vi "Team and Side.vi"(5 "Lado":enum16{"Esquerdo", "Direito"}(ring) caption="Enum", 7 "Time":enum16{"Azul", "Amarelo"}(ring) caption="Enum", 9 "Comm RX FPS":dbl, 10 "Game Status":T17 {"Time" format="%<%.3X %x>T"; "Blue Timeout Remaining" format="%<%M:%S>t"; "Yellow Timeout Remaining" format="%<%M:%S>t"; "Time Left" format="%<%M:%S>t"}, 11 "Field State Input":T1 {"Detection Frame Out"."robots_blue"."height" format="%+4.3f"; "Detection Frame Out"."robots_blue"."pixel_y" format="%+4.3f"; "Detection Frame Out"."robots_blue"."pixel_x" format="%+4.3f"; "Detection Frame Out"."robots_blue"."orientation" format="%+4.3f"; "Detection Frame Out"."robots_blue"."y" format="%+4.3f"; "Detection Frame Out"."robots_blue"."confidence" format="%4.3f"; "Detection Frame Out"."robots_blue"."x" format="%+4.3f"; "Detection Frame Out"."robots_yellow"."height" format="%+4.3f"; "Detection Frame Out"."robots_yellow"."pixel_y" format="%+4.3f"; "Detection Frame Out"."robots_yellow"."pixel_x" format="%+4.3f"; "Detection Frame Out"."robots_yellow"."orientation" format="%+4.3f"; "Detection Frame Out"."robots_yellow"."y" format="%+4.3f"; "Detection Frame Out"."robots_yellow"."confidence" format="%4.3f"; "Detection Frame Out"."robots_yellow"."x" format="%+4.3f"}) -> (3 "IA State":T6={"our_robots"=[], "enemy_robots"=[], "balls"=[], "geometry"={"line_width"=0, "field_length"=0, "field_width"=0, "boundary_width"=0, "referee_width"=0, "goal_width"=0, "goal_depth"=0, "goal_wall_width"=0, "center_circle_radius"=0, "defense_radius"=0, "defense_stretch"=0, "free_kick_from_defense_dist"=0, "penalty_spot_from_field_line_dist"=0, "penalty_line_from_spot_dist"=0}, "IA Judge"={"stage"="", "command"="", "our_goalie_id"=0.0, "enemy_goalie_id"=0.0, "command enum"=enum."Halt", "Time"=enum."Azul"}, "Received Timestamp"=timestamp(0 s since 1904-01-01), "Events"={"Touch"=FALSE, "Ball out"=FALSE, "id touch"=0.0, "Ball out of \nVision"=FALSE, "Ball inside \nGoalie area"=FALSE, "Robot not responding"=FALSE, "Robots responding status"=[1.0, 1.0, 1.0, 1.0, 1.0, 1.0], "Enemy Ball \nPossession"=FALSE, "Pass State"=FALSE, "id end of pass"=0.0, "Kick"=FALSE, "Id ini Possession"=0.0, "Ball Possesion"=FALSE, "Id Possesion"=0.0, "Direct Kick"=FALSE, "2nd Strk Ativo"=FALSE}})   [LabVIEW 2018]
uses:
  SSL Referee Game Status.ctl
  Communication_class/Paths/MessageAI_State Folder/Core/AI Input.ctl
  Controls/AI Robot.ctl
  Controls/Functions Enum.ctl
  Controls/AttackerStates.ctl
  Controls/PathDests.ctl
  Controls/PathDest.ctl
  Communication_class/Paths/MessageAI_State Folder/Core/AI Ball.ctl
  Communication_class/Paths/MessageAI_State Folder/Core/Field Size.ctl
  Communication_class/Paths/MessageAI_State Folder/Core/AI Judge.ctl
  Communication_class/Paths/MessageAI_State Folder/Intel/Command Enum.ctl
  Communication_class/Paths/MessageAI_State Folder/Util/Events/Events.ctl
  Controls/SSL Field State.ctl
  Controls/SSL Detection Frame.ctl
  Controls/SSL Detection Robot.ctl
  <vilib>/Analysis/Matrix/Datatypes/RealMatrix.ctl
  Controls/SSL Detection Ball.ctl
  <vilib>/Analysis/Matrix/NI_Matrix.lvlib
panel:
  # "Score"
  # "Red Cards"
  # "Yellow Cards"
  # "Timeouts Left"
  # "Timeout Remaining"
  # "Goalie ID"
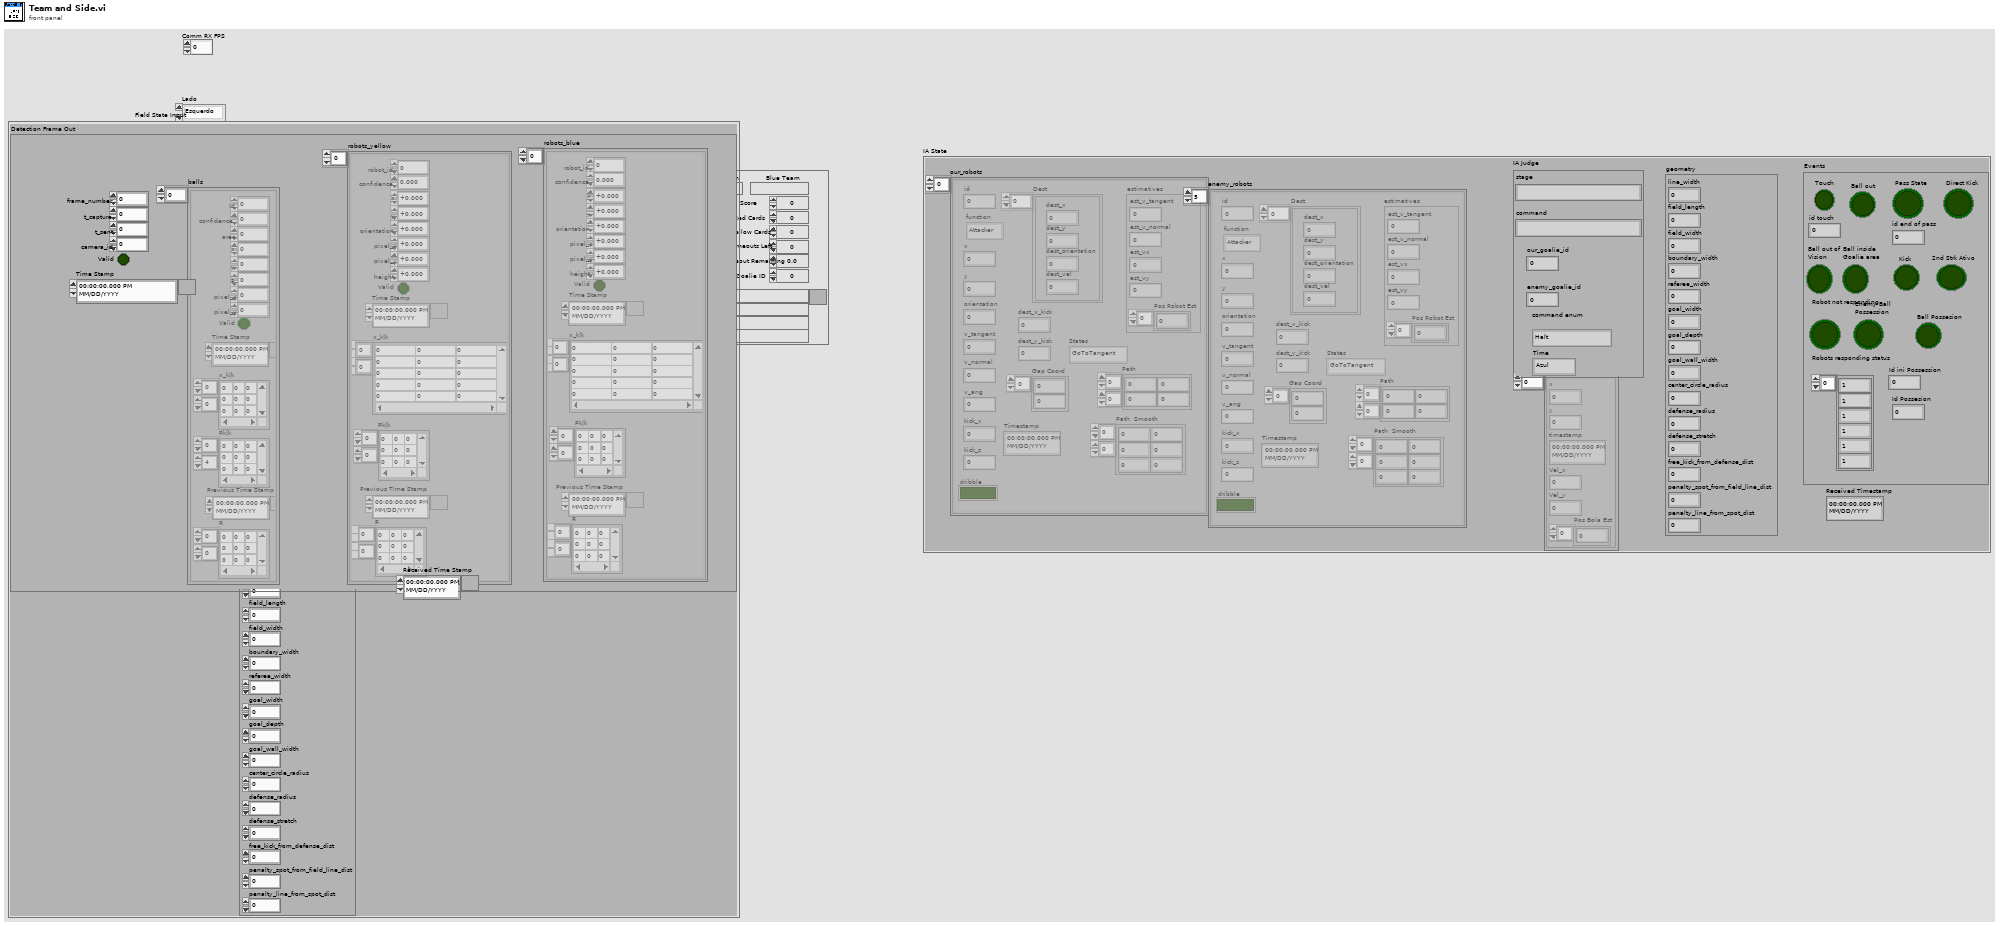
[diagram p1: front panel]
types:
  T1 = typedef "SSL Field State.ctl" = cluster{"Detection Frame Out":T2, "Field Size Out":cluster{"line_width":u32, "field_length":u32, "field_width":u32, "boundary_width":u32, "referee_width":u32, "goal_width":u32, "goal_depth":u32, "goal_wall_width":u32, "center_circle_radius":u32, "defense_radius":u32, "defense_stretch":u32, "free_kick_from_defense_dist":u32, "penalty_spot_from_field_line_dist":u32, "penalty_line_from_spot_dist":u32}, "Received Time Stamp":timestamp}
  T2 = typedef "SSL Detection Frame.ctl" = cluster{"frame_number":u32, "t_capture":dbl, "t_sent":dbl, "camera_id":u32, "robots_yellow":T3[], "robots_blue":T3[], "balls":T5[], "Valid":bool, "Time Stamp":timestamp}
  T3 = typedef "SSL Detection Robot.ctl" = cluster{"x":sgl, "robot_id":u32, "confidence":sgl, "y":sgl, "orientation":sgl, "pixel_x":sgl, "pixel_y":sgl, "height":sgl, "Valid":bool, "Time Stamp":timestamp, "x_k|k":T4, "Pk|k":T4, "Previous Time Stamp":timestamp, "R":T4}
  T4 = typedef "NI_Matrix.lvlib/RealMatrix.ctl" = dbl[][]
  T5 = typedef "SSL Detection Ball.ctl" = cluster{"x":sgl, "area":u32, "confidence":sgl, "y":sgl, "z":sgl, "pixel_x":sgl, "pixel_y":sgl, "Valid":bool, "Time Stamp":timestamp, "x_k|k":T4, "Pk|k":T4, "Id":u32, "Previous Time Stamp":timestamp, "R":T4}
  T6 = typedef "AI Input.ctl" = cluster{"our_robots":T7[], "enemy_robots":T7[], "balls":T12[], "geometry":T13, "IA Judge":T14, "Received Timestamp":timestamp, "Events":T16}
  T7 = typedef "AI Robot.ctl" = cluster{"id":u32, "function":T8, "x":dbl, "y":dbl, "orientation":dbl, "v_tangent":dbl, "v_normal":dbl, "v_ang":dbl, "kick_x":dbl, "kick_z":dbl, "dribble":bool, "Timestamp":timestamp, "estimatives":cluster{"est_v_tangent":dbl, "est_v_normal":dbl, "est_vx":dbl, "est_vy":dbl, "Pos Robot Est":dbl[]}, "dest_x_kick":dbl, "dest_y_kick":dbl, "Gap Coord":dbl[], "States":T9, "Path ":dbl[][], "Path  Smooth":dbl[][], "Dest":T10}
  T8 = typedef "Functions Enum.ctl" = enum16{"2nd Striker", "Attacker", "Goalie", "Defender", "Striker", "Goto 0", "Dummy", "Kicker", "ZigZag 0", "ZigZag 1", "ZigZag 2", "ZigZag 3", "ZigZag 4", "ZigZag 5", "ZigZag 6", "ZigZag 7", "ZigZag 8", ""}
  T9 = typedef "AttackerStates.ctl" = enum16{"Pass", "GoToTangent", "BallGetting", "GoToKick", ""}
  T10 = typedef "PathDests.ctl" = T11[]
  T11 = typedef "PathDest.ctl" = cluster{"dest_x":dbl, "dest_y":dbl, "dest_orientation":dbl, "dest_vel":dbl}
  T12 = typedef "AI Ball.ctl" = cluster{"x":dbl, "y":dbl, "timestamp":timestamp, "Vel_x":dbl, "Vel_y":dbl, "Pos Bola Est":dbl[]}
  T13 = typedef "Field Size.ctl" = cluster{"line_width":u32, "field_length":u32, "field_width":u32, "boundary_width":u32, "referee_width":u32, "goal_width":u32, "goal_depth":u32, "goal_wall_width":u32, "center_circle_radius":u32, "defense_radius":u32, "defense_stretch":u32, "free_kick_from_defense_dist":u32, "penalty_spot_from_field_line_dist":u32, "penalty_line_from_spot_dist":u32}
  T14 = typedef "AI Judge.ctl" = cluster{"stage":string, "command":string, "our_goalie_id":dbl, "enemy_goalie_id":dbl, "command enum":T15, "Time":enum16{"Azul", "Amarelo"}}
  T15 = typedef "Command Enum.ctl" = enum16{"Halt", "Stop", "Force Start", "PKA Normal Start", "Prepare Kickoff Ally", "PKE Normal Start", "Prepare Kickoff Enemy", "Prepare Penalty Ally", "PPA Normal Start", "Prepare Penalty Enemy", "PPE Normal Start", "Direct Free Enemy", "Direct Free Ally", "Indirect Free Enemy", "Indirect Free Ally", "Timeout Enemy", "Timeout Ally", "Goal Enemy", "Goal Ally", "Ball Placement Enemy", "Ball Placement Ally", "Normal Half Time", "Extra Time Break", "Extra Half Time", "None", "Post Game"}
  T16 = typedef "Events.ctl" = cluster{"Touch":bool, "Ball out":bool, "id touch":dbl, "Ball out of \nVision":bool, "Ball inside \nGoalie area":bool, "Robot not responding":bool, "Robots responding status":dbl[], "Enemy Ball \nPossession":bool, "Pass State":bool, "id end of pass":dbl, "Kick":bool, "Id ini Possession":dbl, "Ball Possesion":bool, "Id Possesion":dbl, "Direct Kick":bool, "2nd Strk Ativo":bool}
  T17 = typedef "SSL Referee Game Status.ctl" = cluster{"Stage":string, "Command":string, "Time Left":dbl, "Yellow Team":string, "Blue Team":string, "Yellow Score":u32, "Blue Score":u32, "Yellow Red Cards":u32, "Blue Red Cards":u32, "Yellow Yellow Cards":u32, "Blue Yellow Cards":u32, "Yellow Timeouts Left":u32, "Blue Timeouts Left":u32, "Yellow Timeout Remaining":dbl, "Blue Timeout Remaining":dbl, "Yellow Goalie Id":u32, "Blue Goalie Id":u32, "Time":timestamp}
  T18 = cluster{"line_width":u32, "field_length":u32, "field_width":u32, "boundary_width":u32, "referee_width":u32, "goal_width":u32, "goal_depth":u32, "goal_wall_width":u32, "center_circle_radius":u32, "defense_radius":u32, "defense_stretch":u32, "free_kick_from_defense_dist":u32, "penalty_spot_from_field_line_dist":u32, "penalty_line_from_spot_dist":u32}
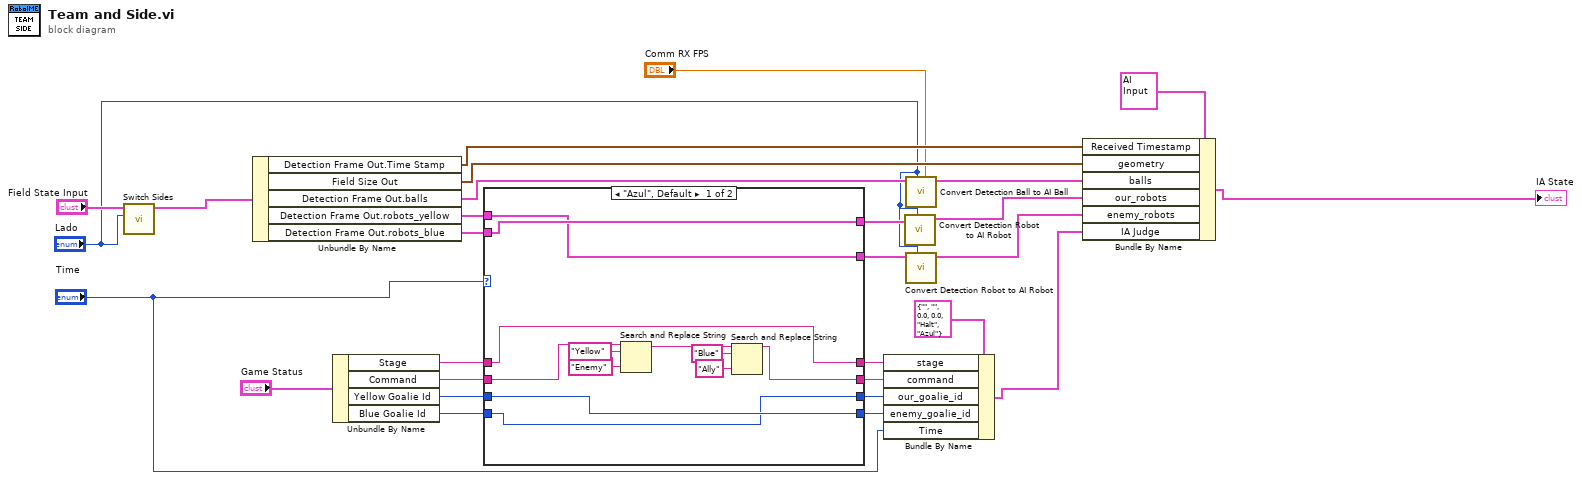
[diagram p0: block diagram]
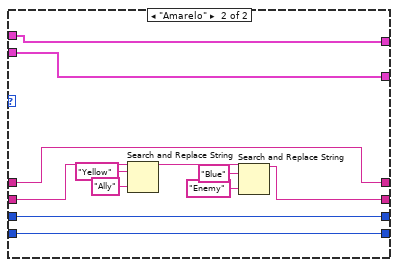
[diagram p2: hidden frame]
diagram:
  n1 = call "Switch Sides.vi"("Lado"="Lado", "Field State Input"="Field State Input") -> ("Field State Side Mirrored"=w27:T1)  [unwired: 9 in]
  n2 = Unbundle By Name(w27) -> ("Detection Frame Out.Time Stamp"=w6:timestamp, "Field Size Out"=w9:T18, "Detection Frame Out.balls"=w10:T5[], "Detection Frame Out.robots_yellow"=w26:T3[], "Detection Frame Out.robots_blue"=w25:T3[])
  n3 = Unbundle By Name("Game Status") -> ("Stage"=w20:string, "Command"=w19:string, "Yellow Goalie Id"=w23:u32, "Blue Goalie Id"=w22:u32)
  n4 = case shown="\"Azul\", Default" "Time" {
    tunnel: w26 -> [w39 w51]
    tunnel: w25 -> [w40 w52]
    tunnel: [w40 w51] -> w14
    tunnel: [w39 w52] -> w12
    tunnel: w23 -> [w38 w50]
    tunnel: w22 -> [w37 w49]
    tunnel: [w38 w49] -> w17
    tunnel: [w37 w50] -> w18
    tunnel: w20 -> [w29 w48]
    tunnel: w19 -> [w31 w47]
    tunnel: [w29 w48] -> w16
    tunnel: [w30 w41] -> w15
    frame "Azul", Default {
      n5 = Search and Replace String(input string=w31, search string="Yellow", replace string="Enemy" ("replace string (\"\")")) -> (result string=w36:string)  [unwired: 5 in, 3 out]
      n6 = Search and Replace String(input string=w36, search string="Blue", replace string="Ally" ("replace string (\"\")")) -> (result string=w30:string)  [unwired: 5 in, 3 out]
    }
    frame "Amarelo" {
      n7 = Search and Replace String(input string=w47, search string="Yellow", replace string="Ally" ("replace string (\"\")")) -> (result string=w42:string)  [unwired: 5 in, 3 out]
      n8 = Search and Replace String(input string=w42, search string="Blue", replace string="Enemy" ("replace string (\"\")")) -> (result string=w41:string)  [unwired: 5 in, 3 out]
    }
  }
  n9 = Bundle By Name(cluster=T14 {"stage"="", "command"="", "our_goalie_id"=0.0, "enemy_goalie_id"=0.0, "command enum"=enum."Halt", "Time"=enum."Azul"} ("IA Judge"), "stage"=w16, "command"=w15, "our_goalie_id"=w18, "enemy_goalie_id"=w17, "Time"="Time") -> (w4:T14)
  n10 = call "Convert Detection Robot to AI Robot.vi"("Lado"="Lado", "Input"=w14) -> ("Output"=w13:T7[])  [unwired: 9 in]
  n11 = call "Convert Detection Ball to AI Ball.vi"("fps"="Comm RX FPS", "Lado"="Lado", "Input"=w10) -> ("Output"=w5:T12[])  [unwired: 8 in]
  n12 = call "Convert Detection Robot to AI Robot.vi"("Lado"="Lado", "Input"=w12) -> ("Output"=w11:T7[])  [unwired: 9 in]
  n13 = Bundle By Name(cluster=T6 {"our_robots"=[], "enemy_robots"=[], "balls"=[], "geometry"={"line_width"=0, "field_length"=0, "field_width"=0, "boundary_width"=0, "referee_width"=0, "goal_width"=0, "goal_depth"=0, "goal_wall_width"=0, "center_circle_radius"=0, "defense_radius"=0, "defense_stretch"=0, "free_kick_from_defense_dist"=0, "penalty_spot_from_field_line_dist"=0, "penalty_line_from_spot_dist"=0}, "IA Judge"={"stage"="", "command"="", "our_goalie_id"=0.0, "enemy_goalie_id"=0.0, "command enum"=enum."Halt", "Time"=enum."Azul"}, "Received Timestamp"=timestamp(0 s since 1904-01-01), "Events"={"Touch"=FALSE, "Ball out"=FALSE, "id touch"=0.0, "Ball out of \nVision"=FALSE, "Ball inside \nGoalie area"=FALSE, "Robot not responding"=FALSE, "Robots responding status"=[1.0, 1.0, 1.0, 1.0, 1.0, 1.0], "Enemy Ball \nPossession"=FALSE, "Pass State"=FALSE, "id end of pass"=0.0, "Kick"=FALSE, "Id ini Possession"=0.0, "Ball Possesion"=FALSE, "Id Possesion"=0.0, "Direct Kick"=FALSE, "2nd Strk Ativo"=FALSE}} ("Detection Frame"), "Received Timestamp"=w6, "geometry"=w9, "balls"=w5, "our_robots"=w13, "enemy_robots"=w11, "IA Judge"=w4) -> (→"IA State":T6)
